vi "Multiple Queued Pedestrian Lights.vi"() -> ()   [LabVIEW 2012]
doc: "Traffic Light VI with the use of Queues and LoadTrafficLightsQueue to Enqueue the Walk Element at the front of the Queue. Has control over both the Traffic Lights display and the Pedestrian Lights Display. Red is set as the initial state.s"
uses:
  Controls/Traffic Light Display.ctl
  Controls/Pedestrian Light Display.ctl
  Controls/Traffic Light States (with Walk State).ctl
panel:
  out "Pedestrian Light Display":T1
  in  "Walk":bool
  in  "Stop Button":bool
  out "Traffic Light Display":T2
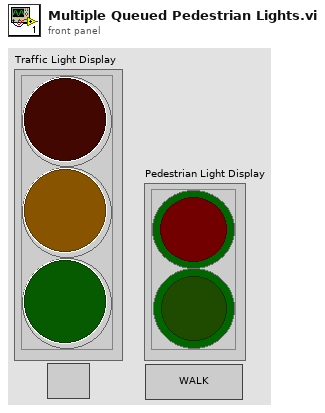
[diagram p1: front panel]
types:
  T1 = typedef "Pedestrian Light Display.ctl" = cluster{"Red":bool, "Green":bool}
  T2 = typedef "Traffic Light Display.ctl" = cluster{"RED":bool, "AMBER":bool, "GREEN":bool}
  T3 = typedef "Traffic Light States (with Walk State).ctl" = enum16{"Red", "RedAmber", "Green", "Amber", "Walk"}
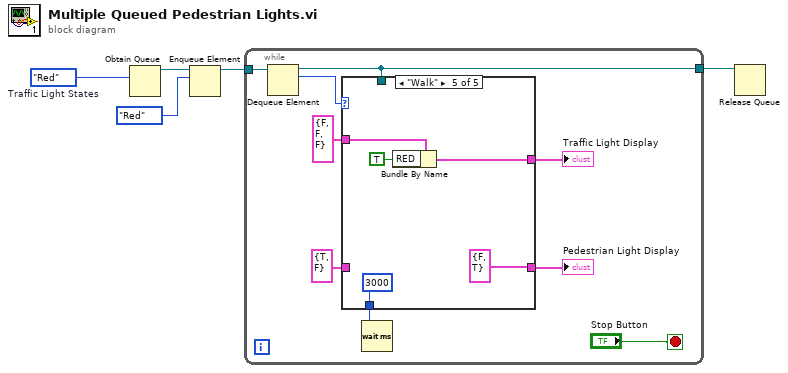
[diagram p0: block diagram]
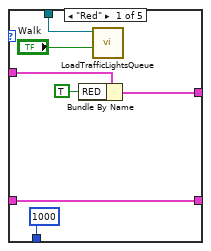
[diagram p2: hidden frame]
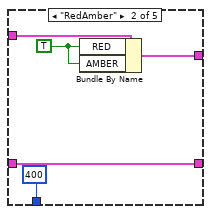
[diagram p3: hidden frame]
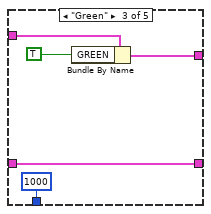
[diagram p4: hidden frame]
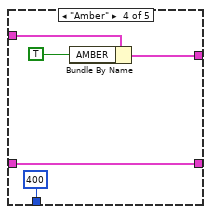
[diagram p5: hidden frame]
diagram:
  w2 = Traffic_Light_States_(with_Walk_State)."Red"  # Traffic Light States
  n1 = Obtain Queue(element data type=w2) -> (queue out=w5:refnum<queue>)  [unwired: 4 in, 2 out]
  n2 = Enqueue Element(queue=w5, element=Traffic_Light_States_(with_Walk_State)."Red" ("Traffic Light States")) -> (queue out=w4:refnum<queue>)  [unwired: 2 in, 2 out]
  n3 = while {
    tunnel: w4 -> [w8]
    tunnel: [w6] -> w3
    stop <- "Stop Button" stop-if-true
    n4 = Dequeue Element(queue=w8) -> (queue out=w6:refnum<queue>, element=w7:T3)  [unwired: 2 in, 2 out]
    n5 = case shown="\"Walk\"" w7 {
      tunnel: T2 {"RED"=FALSE, "AMBER"=FALSE, "GREEN"=FALSE} ("Traffic Light Display") -> [w21 w26 w31 w36 w40]
      tunnel: [w19 w25 w29 w34 w38] -> w13
      tunnel: [1000 400 1000 400 3000] -> w11
      tunnel: T1 {"Red"=TRUE, "Green"=FALSE} ("Pedestrian Light Display") -> [w17 w22 w27 w32 _]
      tunnel: [w17 w22 w27 w32 T1 {"Red"=FALSE, "Green"=TRUE} ("Pedestrian Light Display")] -> w9
      tunnel: w6 -> [w16 _ _ _ _]
      frame "Red" {
        n6 = Bundle By Name(cluster=w21, "RED"=TRUE) -> (w19:T2)
        n7 = call "LoadTrafficLightsQueue.vi"("Queue Ref in"=w16, "Walk"="Walk") -> ()  [unwired: 9 in]
      }
      frame "RedAmber" {
        w24 = TRUE ("RED")
        n8 = Bundle By Name(cluster=w26, "RED"=w24, "AMBER"=w24) -> (w25:T2)
      }
      frame "Green" {
        n9 = Bundle By Name(cluster=w31, "GREEN"=TRUE ("RED")) -> (w29:T2)
      }
      frame "Amber" {
        n10 = Bundle By Name(cluster=w36, "AMBER"=TRUE ("RED")) -> (w34:T2)
      }
      frame "Walk" {
        n11 = Bundle By Name(cluster=w40, "RED"=TRUE) -> (w38:T2)
      }
    }
    "Traffic Light Display" <- w13
    "Pedestrian Light Display" <- w9
    n12 = Wait (ms)(milliseconds to wait=w11) -> ()  [unwired: 1 out]
  }
  n13 = Release Queue(queue=w3) -> ()  [unwired: 2 in, 3 out]
